vi "ReadLine.vi"(8 "error in (no error)":errorcluster, 11 "FTP in":refnum<class "FTP.lvclass">) -> (0 "error out":errorcluster, 1 "Line":string, 2 "code":i32, 3 "FTP out":refnum<class "FTP.lvclass">, 4 "Full Line":string)   [LabVIEW 2020, in "FTP.lvlib" / "FTP.lvclass"]
uses:
  FTP.lvclass
  controls/CmdCluster.ctl
  FTP.lvclass/FTP.ctl
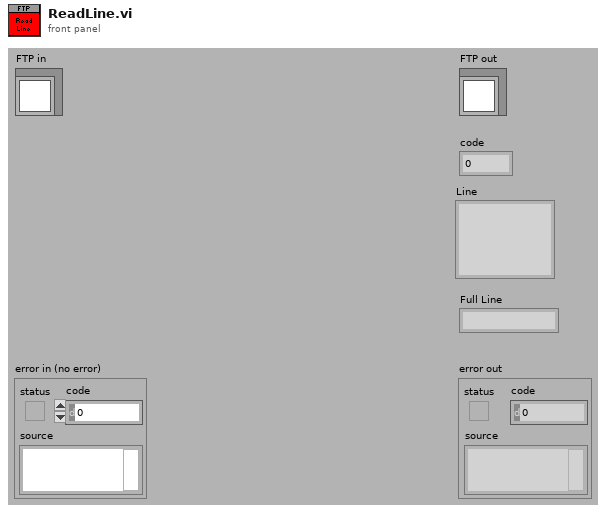
[diagram p1: front panel]
types:
  T1 = typedef "FTP.lvlib/FTP.lvclass/CmdCluster.ctl" = cluster{"CmdSting":string, "FromClient":bool}
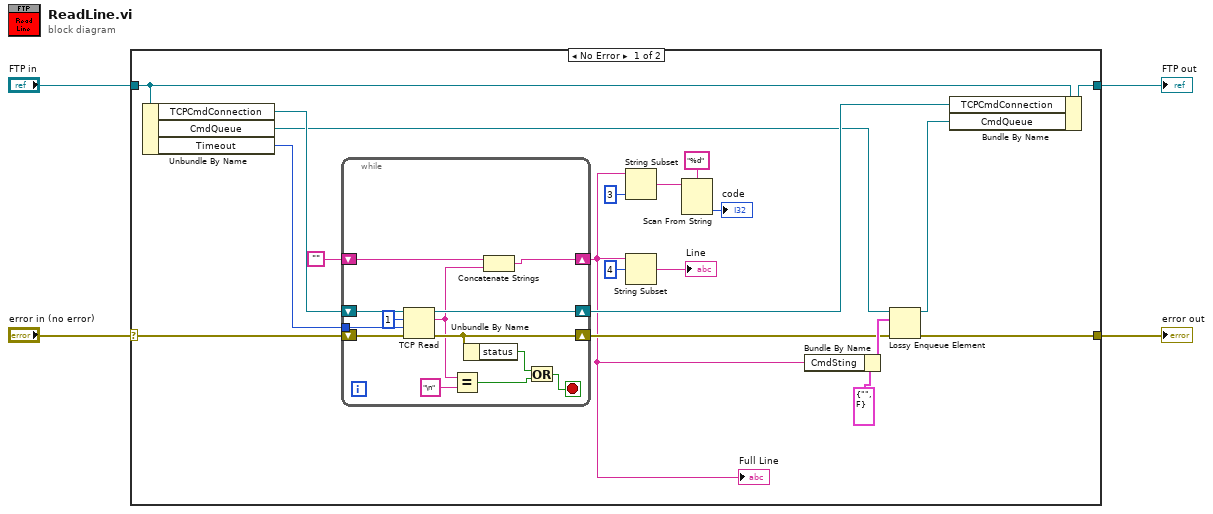
[diagram p0: block diagram]
diagram:
  n1 = case shown="No Error" "error in (no error)" {
    selector: "error in (no error)" -> [w23 w39]
    tunnel: [w13 w39] -> w3
    tunnel: [w22 w38] -> w1
    tunnel: "FTP in" -> [w5 w38]
    frame No Error {
      n2 = Unbundle By Name(w5) -> ("TCPCmdConnection"=w21:refnum<k5>, "CmdQueue"=w15:refnum<queue>, "Timeout"=w6:i32)
      n3 = while {
        shift-right: [w26] -> w7
        shift-left: "" -> [w28]
        shift-right: [w32] -> w8
        shift-left: w23 -> [w37]
        shift-right: [w35] -> w20
        shift-left: w21 -> [w36]
        tunnel: w6 -> [w25]
        stop <- w31 stop-if-true
        n4 = TCP Read(connection ID=w36, bytes to read=1, error in (no error)=w37, 9:w25) -> (connection ID out=w35:refnum<k5>, data out=w27:string, error out=w32:errorcluster)  [unwired: 1 in]
        n5 = Equal?(x=w27, y="\n") -> (x = y?=w29:bool)
        n6 = Unbundle By Name(w32) -> ("status"=w30:bool)
        n7 = Concatenate Strings(w28, w27) -> (w26:string)
        n8 = Or(x=w30, y=w29) -> (x .or. y?=w31:bool)
      }
      "Full Line" <- w7
      n9 = String Subset(string=w7, length (rest)=3 ("length (rest)")) -> (substring=w16:string)  [unwired: 1 in]
      n10 = String Subset(string=w7, offset (0)=4) -> (substring=→"Line":string)  [unwired: 1 in]
      n11 = Scan From String(format string="%d", input string=w16) -> (output 1=→"code":i32)  [unwired: 3 in, 3 out]
      n12 = Bundle By Name(cluster=T1 {"CmdSting"="", "FromClient"=FALSE} ("CmdCluster"), "CmdSting"=w7) -> (w11:T1)
      n13 = Lossy Enqueue Element(queue=w15, element=w11, error in (no error)=w8) -> (queue out=w14:refnum<queue>, error out=w13:errorcluster)  [unwired: 2 out]
      n14 = Bundle By Name(cluster=w5, "TCPCmdConnection"=w20, "CmdQueue"=w14) -> (w22:refnum<class "FTP.lvclass">)
    }
    frame Error {
    }
  }
  "error out" <- w3
  "FTP out" <- w1
